vi "Cryocoller test program.vi"() -> ()   [LabVIEW 2021]
panel:
  out "error out":errorcluster
  out "Raw String Responses":string[](array[string])
  in  "VISA Resource (write)":refnum<visa-resource-name>="COM1"
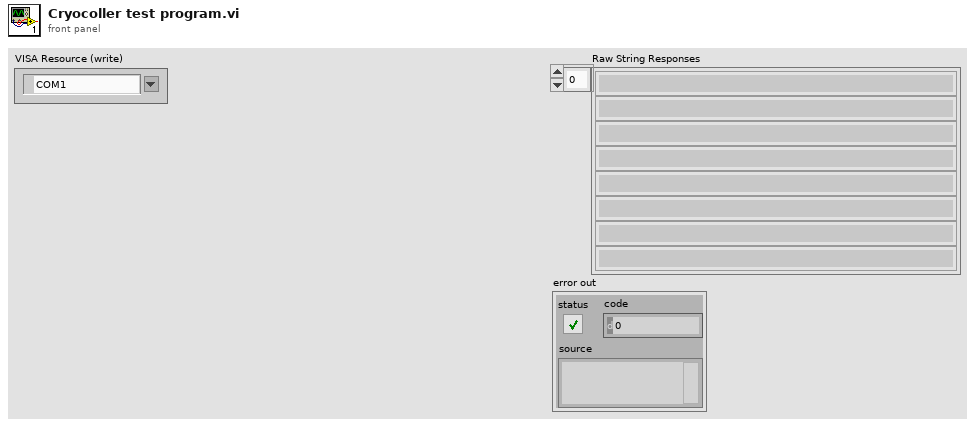
[diagram p1: front panel]
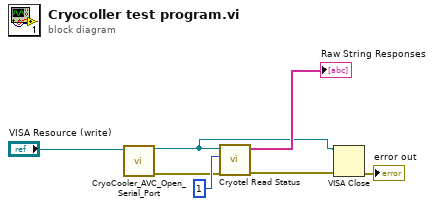
[diagram p0: block diagram]
diagram:
  n1 = call "CryoCooler_AVC_Open_Serial_Port.vi"("VISA Resource (write)"="VISA Resource (write)") -> ("error out"=w6:errorcluster, "VISA Resource out"=w2:refnum<visa-resource-name>)  [unwired: 9 in]
  n2 = call "Cryotel Read Status.vi"("error in"=w6, "Number of reads"=1, "VISA Resource (write)"=w2) -> ("error out"=w3:errorcluster, "Raw String Responses"=→"Raw String Responses":string[])  [unwired: 6 in, 1 out]
  n3 = VISA Close(VISA resource name=w2, error in (no error)=w3) -> (error out=→"error out":errorcluster)
